vi "Parse Partial.vi"(8 "Error In":errorcluster) -> (0 "Error Out":errorcluster)   [LabVIEW 2018, in "Tests.lvlib" / "Lexer.lvlib"]
uses:
  Lexer.lvlib
  src/Toolkit/Low-Level/Tokens/Partial/Partial.lvclass
  src/Toolkit/Low-Level/Tokens/Keyable/Keyable.lvclass/Keyable.ctl
  src/Toolkit/Low-Level/Tokens/Keyable/Read Key.vi
  src/Toolkit/Low-Level/Support/Lex String.vi
  <vilib>/Utility/LVClass/Get LV Class Name.vi
  src/Toolkit/Low-Level/Tokens/Keyable/Keyable.lvclass
  <vilib>/addons/_JKI Toolkits/Caraya/classes/Test/Test.lvclass
  <vilib>/addons/_JKI Toolkits/Caraya/classes/Assert/Assert.lvclass
  Tests.lvlib
  src/Toolkit/Toolkit.lvlib
  src/Toolkit/Low-Level/Tokens/Abstract/Abstract.lvclass
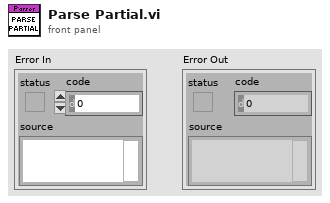
[diagram p1: front panel]
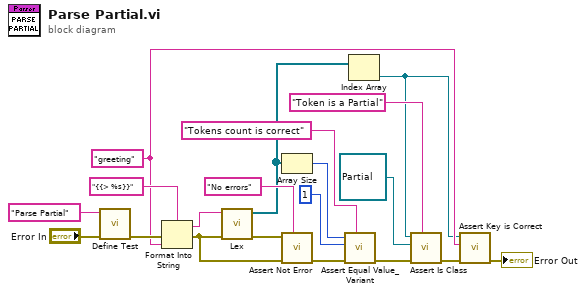
[diagram p0: block diagram]
diagram:
  w5 = "greeting"
  n1 = call <vilib>:"Define Test.vi"("error in (no error)"="Error In", "Label (VI Title)"="Parse Partial") -> ("error out"=w17:errorcluster)  [unwired: 9 in]
  n2 = Format Into String(format string="{{> %s}}", error in=w17, w5) -> (resulting string=w1:string, error out=w2:errorcluster)  [unwired: 1 in]
  n3 = call-poly "Lex.vi"("Error In"=w2, "Input"=w1) -> ("Error Out"=w18:errorcluster, "Tokens"=w11:refnum<class "Abstract.lvclass">[])  [unwired: 8 in]
  n4 = Array Size(array=w11) -> (size(s)=w13:i32)
  n5 = call <vilib>:"Assert Not Error.vi"("Label"="No errors", "error in (no error)"=w2, "Not Error?"=w18) -> ("error out"=w15:errorcluster)  [unwired: 8 in]
  n6 = call <vilib>:"Assert Equal Value_Variant.vi"("Label"="Tokens count is correct", "error in (no error)"=w15, "Y"=1 ("size(s)"), "X"=w13) -> ("error out"=w10:errorcluster)  [unwired: 7 in]
  n7 = Index Array(array=w11) -> (element=w4:refnum<class "Abstract.lvclass">)  [unwired: 1 in]
  n8 = call "Assert Is Class.vi"("Label"="Token is a Partial", "Error In"=w10, "Expected"=refnum<class "Partial.lvclass"> refnum ("Mustache.lvlib:Tokens.lvlib:Partial.lvclass"), "Actual"=w4) -> ("Error Out"=w8:errorcluster)  [unwired: 7 in]
  n9 = call "Assert Key is Correct.vi"("Error In"=w8, "Expected"=w5, "Token"=w4) -> ("Error Out"=→"Error Out":errorcluster)  [unwired: 8 in]
